vi "Operation.vi"(8 "error in (no error)":errorcluster, 10 "operation (meas. mode)":T1=enum."Measurement mode") -> (0 "error out":errorcluster, 2 "return value":i32)   [LabVIEW 2023, in "HighFinesse WS5.lvlib"]
doc: "Sets the operation mode for the wavelength meter. Normally this should be set to \"Measurement mode.\""
uses:
  HighFinesse WS5.lvlib
  Control typedefs.llb/Measurement Mode.ctl
  wlmData.dll
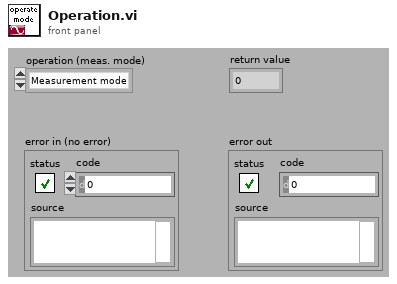
[diagram p1: front panel]
types:
  T1 = typedef "HighFinesse WS5.lvlib/Measurement Mode.ctl" = enum16{"Measurement off", "Adjustment mode", "Measurement mode"}
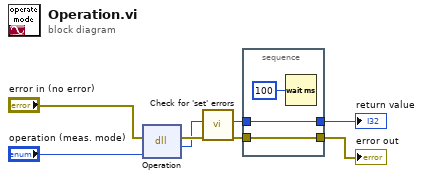
[diagram p0: block diagram]
diagram:
  n1 = dll-call lib="C:/LabVIEW-programs/Instruments/Wavelength meter/HighFinesse WS5/wlmData.dll" fn="Operation"(error in="error in (no error)", "Op"="operation (meas. mode)") -> (error out=w7:errorcluster, "return type"=w6:i32)  [unwired: 2 in, 2 out]
  n2 = call "Check for 'set' errors.vi"("error in (no error)"=w7, "return value"=w6) -> ("error out"=w5:errorcluster, "return value out"=w3:i32)  [unwired: 8 out]
  n3 = stacked-sequence {
    tunnel: w5 -> [w11]
    tunnel: [w11] -> w4
    tunnel: w3 -> [w10]
    tunnel: [w10] -> w1
    frame #0 {
      n4 = Wait (ms)(milliseconds to wait=u32 100) -> ()  [unwired: 1 out]
    }
  }
  "error out" <- w4
  "return value" <- w1
